vi "Start Acquisition and Logging.vi"(8 "error in (no error)":errorcluster, 11 "Acquisition and Logging Configuration":T2={"Samples per Read"=1, "Number of Channels"=12, "Channel Scale Array"=[0.0, 0.0, 0.0, 0.0], "Channel Names"=[], "Trigger - RMS Value"=0.0, "Trigger - Channel"=4, "Trigger - Time (Minute)"=0, "Data Rate"=0, "# Samples After Trigger"=300005, "Thresholds"=[], "Input active"=[]}) -> (0 "error out":errorcluster, 1 "Wait on IRQ Timeout?":bool, 3 "FPGA VI Reference":T1)   [LabVIEW 2014]
uses:
  controls/Acquisition and Logging Configuration.ctl
  controls/FPGA VI Reference.ctl
  <vilib>/FPGAPlugInAG/cRIO-9114/niLvFpga_Open_cRIO-9114.vi
  <vilib>/rvi/interface/common/dynamic/niFpgaDynamicAddResources.vi
  <vilib>/FPGAPlugInAG/Dynamic/niLvFpga_Reset_Dynamic.vi
  <vilib>/Utility/error.llb/Error Cluster From Error Code.vi
  <vilib>/rvi/errors/niLvFpgaAdjustHostInterfaceError.vi
  <vilib>/rvi/interface/common/niFpgaWaitOnOcc.vi
  <vilib>/FPGAPlugInAG/Dynamic/niLvFpga_Run_Dynamic.vi
  <vilib>/RVI Host/nirviSupport.llb/nirviErrorClusterFromErrorCode.vi
  <vilib>/rvi/interface/nirviOpenFPGA/nirviOpenFPGA.xnode
  FPGA Bitfiles/FreiaInterlock_FPGATarget_FPGAMain_d9emsL9JL5U.lvbitx
  FPGA Main.vi
  <vilib>/rvi/interface/nirviMethod/nirviMethod.xnode
  <vilib>/rvi/interface/nirviReadWriteControl/nirviReadWriteControl.xnode
  <vilib>/rvi/errors/niLvFpgaMergeErrorWithErrorCode.vi
  <vilib>/rvi/interface/nirviMethod/StockFPGA_InlinedMethodWaitForSingleIRQ.vi
  <vilib>/FPGAPlugInAG/Dynamic/niLvFpga_WaitOnIrq_Dynamic.vi
  <vilib>/FPGAPlugInAG/Dynamic/niLvFpga_AcknowledgeIrq_Dynamic.vi
  <vilib>/FPGAPlugInAG/Dynamic/niLvFpga_ConfigureFifo_Dynamic.vi
  <vilib>/FPGAPlugInAG/Dynamic/niLvFpga_StartFifo_Dynamic.vi
  NiFpgaLv.dll
  <vilib>/rvi/interface/Simulation/niFpgaSimulationCallBeginRW.vi
panel:
  out "Actual Depth":u32
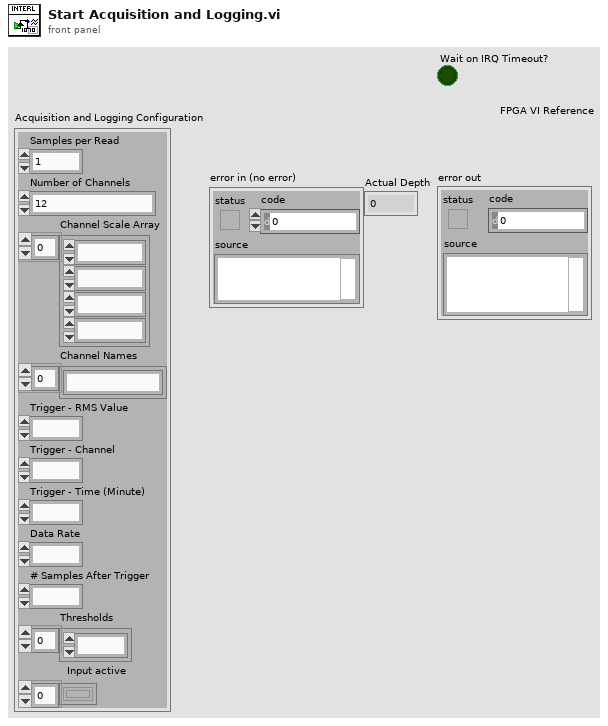
[diagram p1: front panel]
types:
  T1 = typedef "FPGA VI Reference.ctl" = refnum<k20>
  T2 = typedef "Acquisition and Logging Configuration.ctl" = cluster{"Samples per Read":i32, "Number of Channels":u32, "Channel Scale Array":fxp<+,24,12>[], "Channel Names":string[], "Trigger - RMS Value":dbl, "Trigger - Channel":i32, "Trigger - Time (Minute)":i32, "Data Rate":i32, "# Samples After Trigger":u32, "Thresholds":dbl[], "Input active":bool[]}
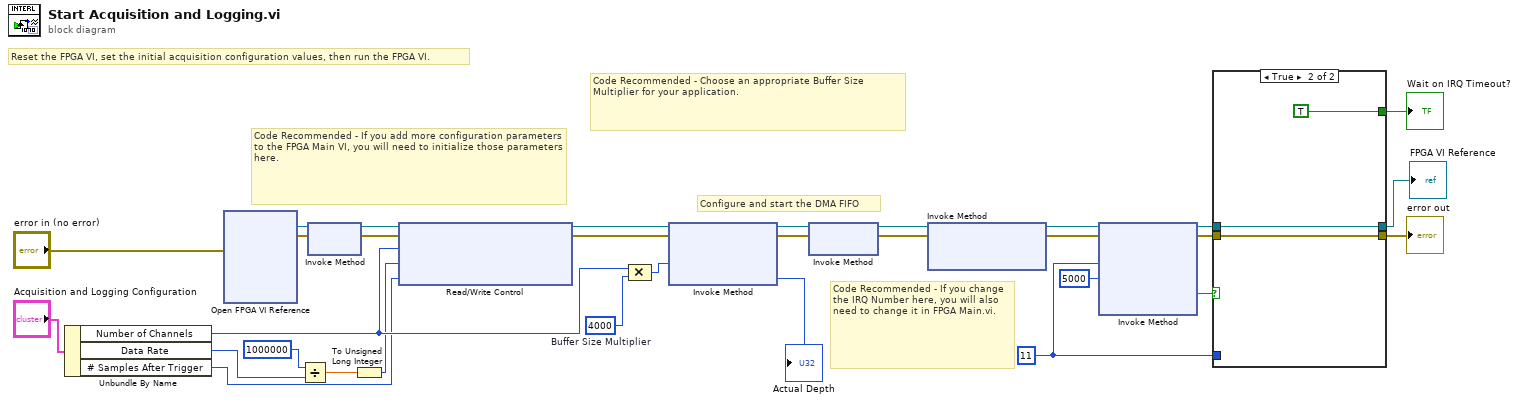
[diagram p0: block diagram]
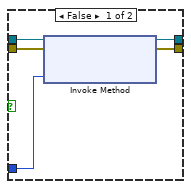
[diagram p2: hidden frame]
diagram:
  w12 = 11
  w13 = 4000  # Buffer Size Multiplier
  # "Code Recommended - If you change the IRQ Number here, you will also need to change it in FPGA Main.vi."
  # "Code Recommended - Choose an appropriate Buffer Size Multiplier for your application."
  # "Configure and start the DMA FIFO"
  # "Code Recommended - If you add more configuration parameters to the FPGA Main VI, you will need to initialize those parameters here."
  # "Reset the FPGA VI, set the initial acquisition configuration values, then run the FPGA VI."
  n1 = Unbundle By Name("Acquisition and Logging Configuration") -> ("Number of Channels"=w14:u32, "Data Rate"=w6:i32, "# Samples After Trigger"=w1:u32)
  n2 = xnode "Open FPGA VI Reference"("error in"="error in (no error)") -> ("FPGA VI Reference Out"=w11:refnum<k20>, "error out"=w10:errorcluster)  [unwired: 1 in]
  n3 = Divide(x=1000000 ("y"), y=w6) -> (x/y=w3:dbl)
  n4 = xnode "Invoke Method"("FPGA VI Reference In"=w11, "error in"=w10) -> ("FPGA VI Reference Out"=w29:refnum<k20>, "error out"=w28:errorcluster)
  n5 = To Unsigned Long Integer(number=w3) -> (unsigned 32bit integer=w4:u32)
  n6 = xnode "Read/Write Control"("FPGA VI Reference In"=w29, "error in"=w28, "Number of Channels"=w14, "Sample Period (uSec)"=w4, "Number samples after trigger"=w1) -> ("FPGA VI Reference Out"=w16:refnum<k20>, "error out"=w15:errorcluster)
  n7 = Compound Arithmetic op=MULTIPLY(w14, w13) -> (w8:u32)
  n8 = xnode "Invoke Method"("FPGA VI Reference In"=w16, "error in"=w15, "Requested Depth"=w8) -> ("FPGA VI Reference Out"=w19:refnum<k20>, "error out"=w20:errorcluster, "Actual Depth"=→"Actual Depth":u32)
  n9 = xnode "Invoke Method"("FPGA VI Reference In"=w19, "error in"=w20) -> ("FPGA VI Reference Out"=w17:refnum<k20>, "error out"=w18:errorcluster)
  n10 = xnode "Invoke Method"("FPGA VI Reference In"=w17, "error in"=w18) -> ("FPGA VI Reference Out"=w30:refnum<k20>, "error out"=w31:errorcluster)  [unwired: 1 in]
  n11 = xnode "Invoke Method"("FPGA VI Reference In"=w30, "error in"=w31, "IRQ Number(s)"=w12, "Timeout (ms)"=5000) -> ("FPGA VI Reference Out"=w22:refnum<k20>, "error out"=w23:errorcluster, "Timed Out"=w25:bool)  [unwired: 1 out]
  n12 = case shown="True" w25 {
    tunnel: w22 -> [w36 w37]
    tunnel: w23 -> [w35 w39]
    tunnel: [w34 w39] -> w26
    tunnel: w12 -> [w33 _]
    tunnel: [_ TRUE] -> w27
    tunnel: [w32 w37] -> w2
    frame False {
      n13 = xnode "Invoke Method"("FPGA VI Reference In"=w36, "error in"=w35, "IRQ Number(s)"=w33) -> ("FPGA VI Reference Out"=w32:refnum<k20>, "error out"=w34:errorcluster)
    }
    frame True {
    }
  }
  "Wait on IRQ Timeout?" <- w27
  "error out" <- w26
  "FPGA VI Reference" <- w2
